vi "Write to EEPROM.vi"(8 "error in (no error)":errorcluster, 9 "15 Byte ASCII":string, 10 "EEPROM Index":u8, 11 "VISA resource name":refnum<visa-resource-name>) -> (0 "error out":errorcluster, 3 "VISA resource name out":refnum<visa-resource-name>)   [LabVIEW 2012, in "Ocean Optics 2000 4000.lvlib"]
doc: "Writes ASCII data to the specific address of the spectrometer EEPROM."
uses:
  Ocean Optics 2000 4000.lvlib
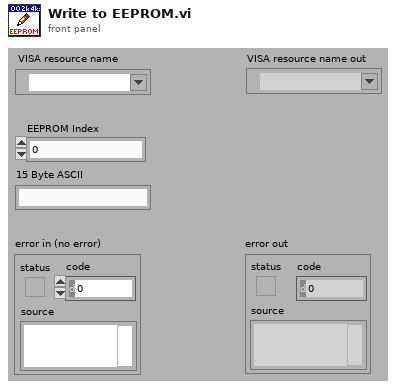
[diagram p1: front panel]
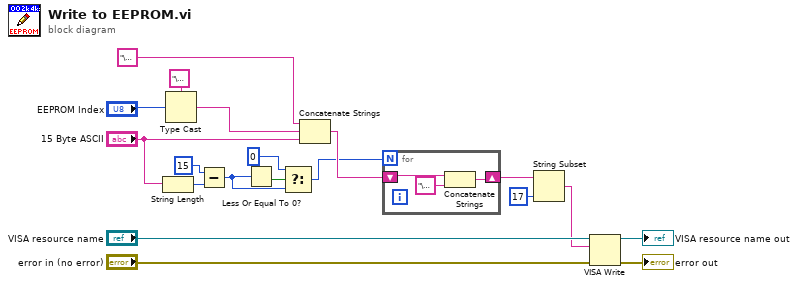
[diagram p0: block diagram]
diagram:
  n1 = String Length(string="15 Byte ASCII") -> (length=w19:i32)
  n2 = Type Cast(type="\u0000", x="EEPROM Index") -> (*(type *) &x=w14:string)
  n3 = Subtract(x=15, y=w19) -> (x-y=w8:i32)
  n4 = Less Or Equal To 0?(x=w8) -> (x <= 0?=w11:bool)
  n5 = Select(t=0, s=w11, f=w8) -> (s? t:f=w9:i32)
  n6 = Concatenate Strings("\u0006" ("string"), w14, "15 Byte ASCII") -> (w12:string)
  n7 = for {
    N: w9 -> [_]
    shift-right: [w21] -> w7
    shift-left: w12 -> [w22]
    n8 = Concatenate Strings(w22, "\u0000" ("string")) -> (w21:string)
  }
  n9 = String Subset(string=w7, length (rest)=17 ("length (rest)")) -> (substring=w3:string)  [unwired: 1 out]
  n10 = VISA Write(VISA resource name="VISA resource name", write buffer=w3, error in (no error)="error in (no error)") -> (VISA resource name out=→"VISA resource name out":refnum<visa-resource-name>, error out=→"error out":errorcluster)  [unwired: 1 out]
